vi "Overlay Access Scope Test.vi"() -> ()   [LabVIEW 2020, in "VI Properties Editor.lvlib"]
uses:
  VI Properties Editor.lvlib
panel:
  out "new picture":picture
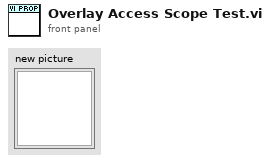
[diagram p1: front panel]
types:
  T1 = typedef "imagedata.ctl" = cluster{"image type":i32, "image depth":i32, "image":u8[], "mask":u8[], "colors":u32[], "Rectangle":cluster{"left":i16, "top":i16, "right":i16, "bottom":i16}}
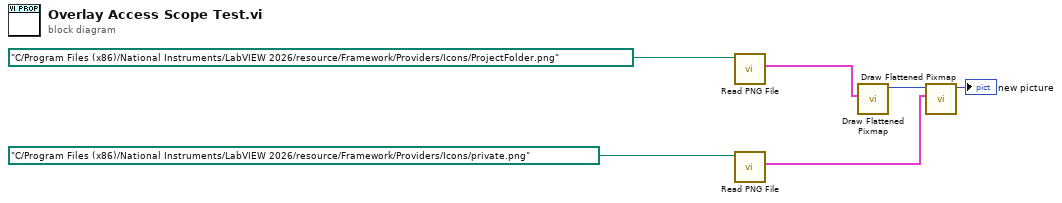
[diagram p0: block diagram]
diagram:
  n1 = call <vilib>:"Read PNG File.vi"("path to PNG file"=path "C:/Program Files (x86)/National Instruments/LabVIEW 2026/resource/Framework/Providers/Icons/ProjectFolder.png") -> ("image data"=w4:T1)  [unwired: 8 in, 2 out]
  n2 = call <vilib>:"Read PNG File.vi"("path to PNG file"=path "C:/Program Files (x86)/National Instruments/LabVIEW 2026/resource/Framework/Providers/Icons/private.png") -> ("image data"=w2:T1)  [unwired: 8 in, 2 out]
  n3 = call <vilib>:"Draw Flattened Pixmap.vi"("image data"=w4) -> ("new picture"=w3:picture)  [unwired: 8 in]
  n4 = call <vilib>:"Draw Flattened Pixmap.vi"("image data"=w2, "picture"=w3) -> ("new picture"=→"new picture":picture)  [unwired: 7 in]
